vi "JSON TO NUMBER_PRESSURE.vi"(7 "IP":string="192.168.23.100", 8 "error in (no error)":errorcluster, 10 "PORT":dbl=1.0 min=1.0 max=4.0 step=1.0, 11 "MASTER":dbl=1.0 min=1.0 max=10.0 step=1.0) -> (0 "error out":errorcluster, 3 "Pressure":dbl format="%#_g bar")   [LabVIEW 2022 SP3]
uses:
  <vilib>/JDP Science/JSONtext/JSONtext.lvlib
panel:
  out "JSON PCK":string
  out "Switching output":i32
  out "/Scale":i32
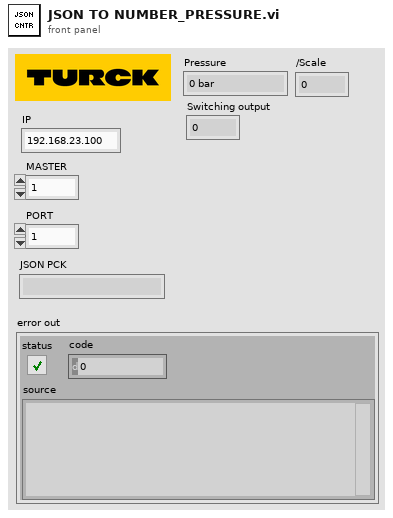
[diagram p1: front panel]
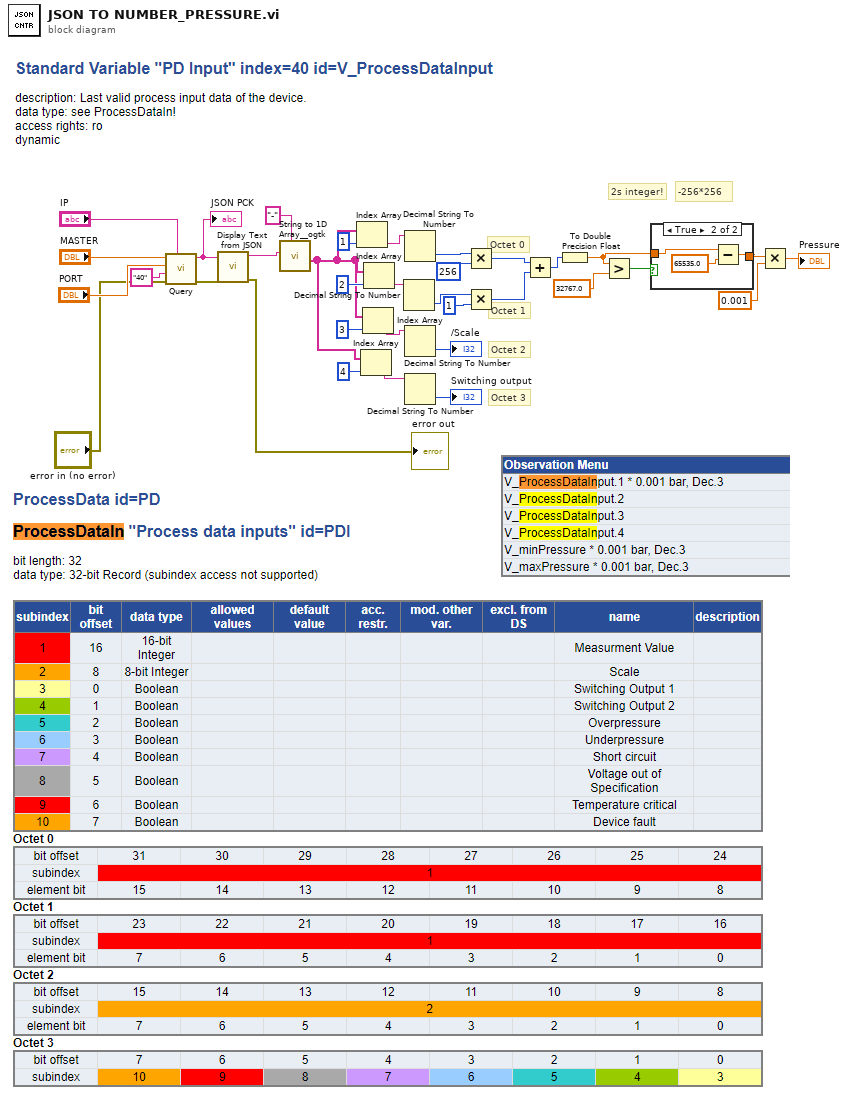
[diagram p0: block diagram]
diagram:
  # "-256*256"
  # "2s integer!"
  # "Octet 3"
  # "Octet 2"
  # "Octet 1"
  # "Octet 0"
  n1 = call "Query.vi"("IP"="IP", "error in (no error)"="error in (no error)", "PARAMETERS"="40", "PORT"="PORT", "MASTER"="MASTER") -> ("error out"=w12:errorcluster, "Response"=w34:string)  [unwired: 5 in]
  "JSON PCK" <- w34
  n2 = call <vilib>:"Display Text from JSON.vi"("error in (no error)"=w12, "Input JSON"=w34) -> ("error out"=→"error out":errorcluster, "Display Text"=w17:string)  [unwired: 7 in, 1 out]
  n3 = call <userlib>:"String to 1D Array__ogtk.vi"("delimiter (Tab)"="-", "string"=w17) -> ("Array of Strings"=w27:string[])  [unwired: 9 in]
  n4 = Index Array(array=w27, index=1) -> (element=w18:string)
  n5 = Index Array(array=w27, index=4) -> (element=w21:string)
  n6 = Index Array(array=w27, index=3) -> (element=w20:string)
  n7 = Index Array(array=w27, index=2) -> (element=w19:string)
  n8 = Decimal String To Number(string=w19) -> (number=w22:i32)  [unwired: 2 in, 1 out]
  n9 = Decimal String To Number(string=w18) -> (number=w16:i32)  [unwired: 2 in, 1 out]
  n10 = Decimal String To Number(string=w20) -> (number=→"/Scale":i32)  [unwired: 2 in, 1 out]
  n11 = Decimal String To Number(string=w21) -> (number=→"Switching output":i32)  [unwired: 2 in, 1 out]
  n12 = Multiply(x=w16, y=u32 256) -> (x*y=w8:u32)
  n13 = Multiply(x=w22, y=u32 1) -> (x*y=w9:u32)
  n14 = Add(x=w8, y=w9) -> (x+y=w7:u32)
  n15 = To Double Precision Float(number=w7) -> (double precision float=w4:dbl)
  n16 = Greater?(x=w4, y=32767.0) -> (0:w6:bool)
  n17 = case shown="True" w6 {
    tunnel: [w35 w38] -> w3
    tunnel: w4 -> [w35 w36]
    frame False {
    }
    frame True {
      n18 = Subtract(x=w36, y=65535.0) -> (x-y=w38:dbl)
    }
  }
  n19 = Multiply(x=w3, y=0.001) -> (x*y=→"Pressure":dbl)
